vi "RobotDriveOpen4MotorWithTalonSRXCAN.vi"(0 "Rear Left Motor":u8=20, 1 "Rear Left Motor Inverted":bool, 2 "Rear Right Motor Inverted":bool, 5 "Rear Right Motor":u8=20, 7 "Front Left Motor":u8=20, 9 "Front Right Motor":u8=20, 11 "error in (no error)":errorcluster, 12 "Front Left Motor Inverted":bool, 13 "Front Right Motor Inverted":bool) -> (4 "RobotDriveDevRef":T1={"DevStatus"={"status"=FALSE, "code"=0, "source"=""}, "Motors[]"=[], "Square Inputs"=FALSE, "Max Output"=1.0}, 15 "error out":errorcluster)   [LabVIEW 2017]
doc: "Opens a reference to the robot drive for a four-motor robot using TalonSRX motor controllers.\n\nThis software is licensed. Open the labview\\readme\\WPI Robotics Library Open Source License.txt file for more information."
uses:
  <vilib>/Rock Robotics/WPI/RobotDrive/WPI_RobotDriveDevRef.ctl
  <vilib>/Rock Robotics/SystemInterfaces/DIO/FPGA_DIOPWMChannel.ctl
  <vilib>/Rock Robotics/WPI/PWM/WPI_PWMDeadband.ctl
  <vilib>/Rock Robotics/WPI/SafetyOutput/WPI_SafetyOutputConfigMenu.ctl
  <vilib>/Rock Robotics/WPI/MotorControl/WPI_MotorControlDeviceRef.ctl
  <vilib>/Rock Robotics/WPI/MotorControl/WPI_MotorControlType.ctl
  <vilib>/Rock Robotics/WPI/ThirdParty/CanMotor/TalonSRX/WPI_CANTalonSRX_APIControlMode.ctl
  <vilib>/Rock Robotics/SystemInterfaces/DIO/FPGA_DIOChannel.ctl
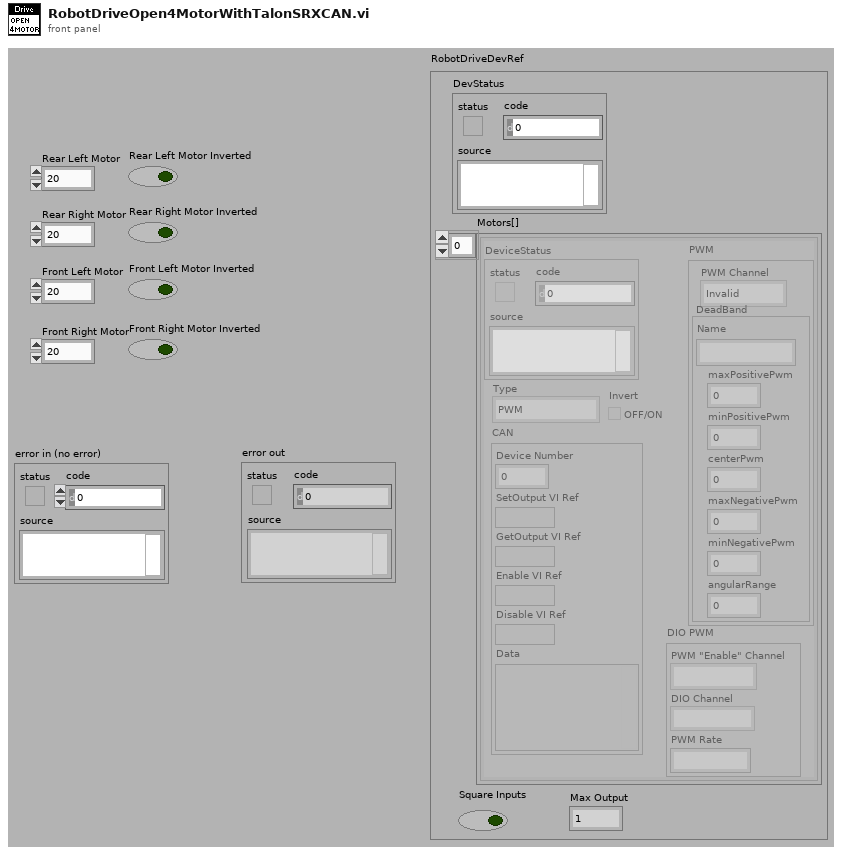
[diagram p1: front panel]
types:
  T1 = typedef "WPI_RobotDriveDevRef.ctl" = cluster{"DevStatus":errorcluster, "Motors[]":T2[], "Square Inputs":bool, "Max Output":dbl}
  T2 = typedef "WPI_MotorControlDeviceRef.ctl" = cluster{"DeviceStatus":errorcluster, "Type":T3, "PWM":cluster{"PWM Channel":T4, "DeadBand":T5}, "CAN":cluster{"Device Number":u8, "SetOutput VI Ref":variant, "GetOutput VI Ref":variant, "Enable VI Ref":variant, "Disable VI Ref":variant, "Data":variant}, "Invert":bool, "DIO PWM":cluster{"PWM \"Enable\" Channel":T4, "DIOChannel":T6, "PWM Rate":dbl}}
  T3 = typedef "WPI_MotorControlType.ctl" = enum16{"PWM", "CAN", "DIO PWM"}
  T4 = typedef "FPGA_DIOPWMChannel.ctl" = enum8{"PWM 0", "PWM 1", "PWM 2", "PWM 3", "PWM 4", "PWM 5", "PWM 6", "PWM 7", "PWM 8", "PWM 9", "PWM MXP 0", "PWM MXP 1", "PWM MXP 2", "PWM MXP 3", "PWM MXP 4", "PWM MXP 5", "PWM MXP 6", "PWM MXP 7", "PWM MXP 8", "PWM MXP 9", "Invalid"}
  T5 = typedef "WPI_PWMDeadband.ctl" = cluster{"Name":string, "maxPositivePwm":i32, "minPositivePwm":i32, "centerPwm":i32, "maxNegativePwm":i32, "minNegativePwm":i32, "angularRange":u16}
  T6 = typedef "FPGA_DIOChannel.ctl" = enum8{"DIO 0", "DIO 1", "DIO 2", "DIO 3", "DIO 4", "DIO 5", "DIO 6", "DIO 7", "DIO 8", "DIO 9", "DIO MXP 0", "DIO MXP 1", "DIO MXP 2", "DIO MXP 3", "DIO MXP 4", "DIO MXP 5", "DIO MXP 6", "DIO MXP 7", "DIO MXP 8", "DIO MXP 9", "DIO MXP 10", "DIO MXP 11", "DIO MXP 12", "DIO MXP 13", "DIO MXP 14", "DIO MXP 15", "SPI Port CS1", "SPI Port CS2", "SPI Port CS3", "SPI Port MISO", "SPI Port MOSI", "Invalid"}
  T7 = typedef "WPI_SafetyOutputConfigMenu.ctl" = enum16{"Enable", "Disable"}
  T8 = typedef "WPI_CANTalonSRX_APIControlMode.ctl" = enum8{"Percent VBus", "Speed", "Position", "Slave", "Unchanged / Invalid", "Voltage Compensation", "Current", "Motion Profile", "Motion Magic"}
  T9 = typedef "WPI_MotorControlDeviceRef.ctl" = cluster{"DeviceStatus":errorcluster, "Type":T10, "PWM":cluster{"PWM Channel":T4, "DeadBand":T5}, "CAN":cluster{"Device Number":u8, "SetOutput VI Ref":variant, "GetOutput VI Ref":variant, "Enable VI Ref":variant, "Disable VI Ref":variant, "Data":variant}, "Invert":bool}
  T10 = typedef "WPI_MotorControlType.ctl" = enum16{"PWM", "CAN"}
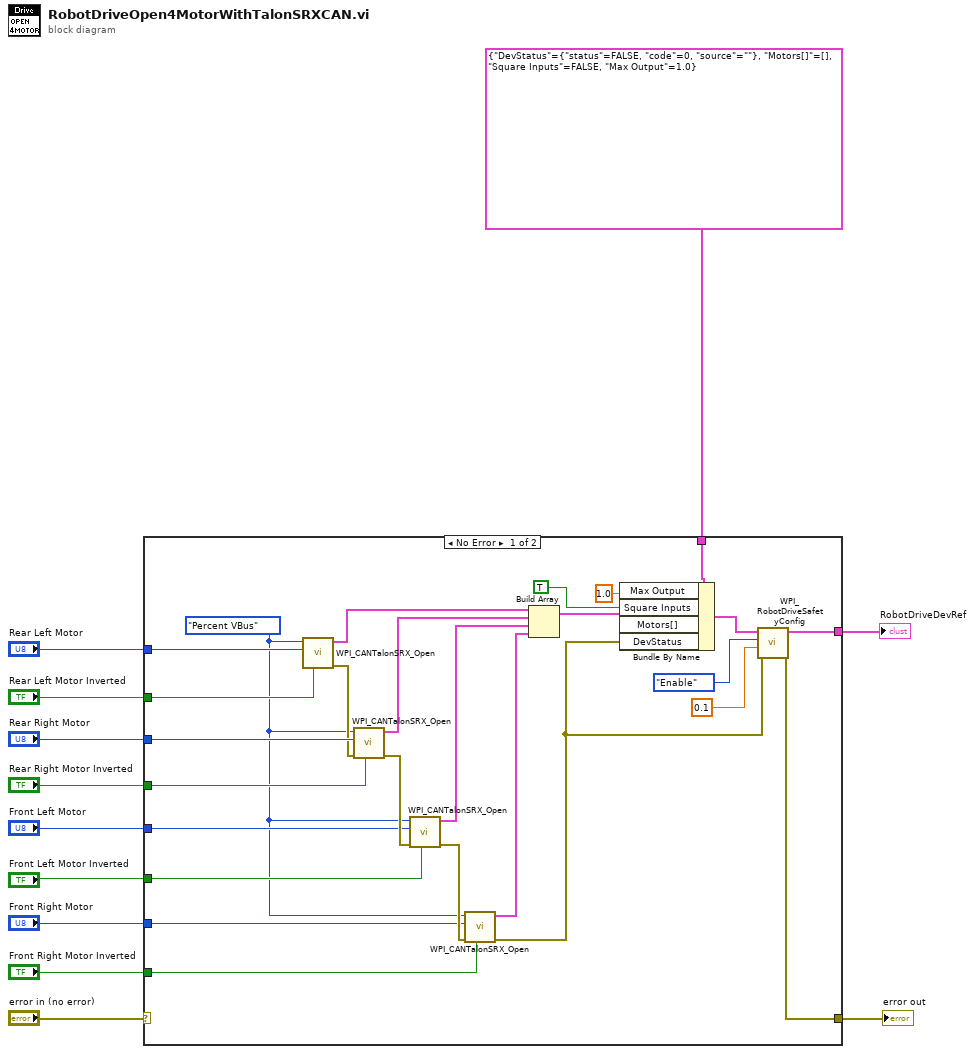
[diagram p0: block diagram]
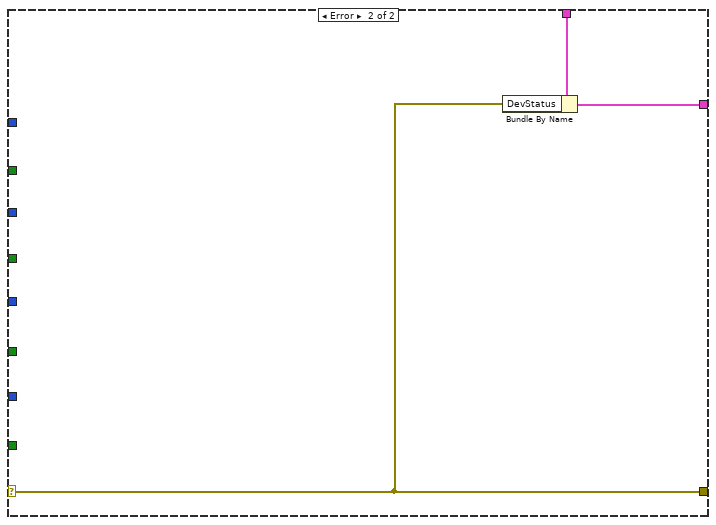
[diagram p2: hidden frame]
diagram:
  n1 = case shown="No Error" "error in (no error)" {
    selector: "error in (no error)" -> [_ w39]
    tunnel: [w23 w40] -> w12
    tunnel: T1 {"DevStatus"={"status"=FALSE, "code"=0, "source"=""}, "Motors[]"=[], "Square Inputs"=FALSE, "Max Output"=1.0} ("RobotDriveDevRef") -> [w38 w41]
    tunnel: "Rear Left Motor" -> [w14 _]
    tunnel: "Front Right Motor" -> [w20 _]
    tunnel: "Front Left Motor" -> [w19 _]
    tunnel: "Rear Right Motor" -> [w18 _]
    tunnel: "Rear Left Motor Inverted" -> [w15 _]
    tunnel: "Rear Right Motor Inverted" -> [w30 _]
    tunnel: "Front Right Motor Inverted" -> [w28 _]
    tunnel: "Front Left Motor Inverted" -> [w29 _]
    tunnel: [w24 w39] -> w1
    frame No Error {
      w13 = WPI_CANTalonSRX_APIControlMode."Percent VBus" ("Control Mode")
      n2 = call <vilib>:"WPI_CANTalonSRX_Open.vi"("Invert"=w15, "Device Number"=w14, "Control Mode"=w13) -> ("error out"=w16:errorcluster, "CAN Talon SRX Ref"=w17:T9)  [unwired: 7 in]
      n3 = call <vilib>:"WPI_CANTalonSRX_Open.vi"("Invert"=w30, "error in"=w16, "Device Number"=w18, "Control Mode"=w13) -> ("error out"=w32:errorcluster, "CAN Talon SRX Ref"=w36:T9)  [unwired: 6 in]
      n4 = call <vilib>:"WPI_CANTalonSRX_Open.vi"("Invert"=w29, "error in"=w32, "Device Number"=w19, "Control Mode"=w13) -> ("error out"=w33:errorcluster, "CAN Talon SRX Ref"=w35:T9)  [unwired: 6 in]
      n5 = call <vilib>:"WPI_CANTalonSRX_Open.vi"("Invert"=w28, "error in"=w33, "Device Number"=w20, "Control Mode"=w13) -> ("error out"=w25:errorcluster, "CAN Talon SRX Ref"=w34:T9)  [unwired: 6 in]
      n6 = Build Array(w17, w36, w35, w34) -> (w31:T9[])
      n7 = Bundle By Name(cluster=w38, "Max Output"=1.0, "Square Inputs"=TRUE ("DestroyPWM?"), "Motors[]"=w31, "DevStatus"=w25) -> (w26:T1)
      n8 = call <vilib>:"WPI_RobotDriveSafetyConfig.vi"("error in (no error)"=w25, "timeout (s)"=0.1, "mode"=WPI_SafetyOutputConfigMenu."Enable", "RobotDriveDevRef"=w26) -> ("error out"=w24:errorcluster, "RobotDriveDevRef"=w23:T1)  [unwired: 6 out]
    }
    frame Error {
      n9 = Bundle By Name(cluster=w41, "DevStatus"=w39) -> (w40:T1)
    }
  }
  "RobotDriveDevRef" <- w12
  "error out" <- w1
